vi "_Beep_Button.vi"(4 "状态输入":bool) -> (1 "状态输出":bool)   [LabVIEW 2020, in "Beep.lvlib"]
uses:
  Beep.lvlib
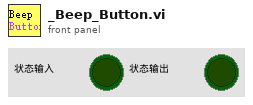
[diagram p1: front panel]
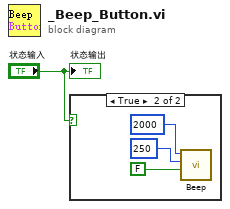
[diagram p0: block diagram]
diagram:
  n1 = case shown="True" "状态输入" {
    frame False {
    }
    frame True {
      n2 = call <vilib>:"Beep.vi"("use system alert? (T)"=FALSE, "duration (msec)"=250, "frequency (Hz)"=2000) -> ()  [unwired: 9 in]
    }
  }
  "状态输出" <- "状态输入"
